vi "niDTS WLAN Rx Test UTIL Static Default Parameters.vi"(10 "Standard":T2 caption="802.11 Standard") -> (2 "Static Default Parameters":T1={"Standard"=enum."802.11 n HT", "DSSS Data Rate (Mbps)"=enum."1", "OFDM Data Rate (Mbps)"=enum."54", "MCS Index"=7, "N Spatial Streams"=1, "Chains"=[TRUE, FALSE, FALSE, FALSE], "Bandwidth (Hz)"=enum."20 MHz", "Channel"=1, "Power (dBm)"=0.0, "Guard Interval"=enum."SHORT", "FEC Coding"=enum."LDPC", "16 symbols"=TRUE, "Payload Length (bytes)"=1500, "Idle Interval (s)"=0.0001, "External Attenuation (dB)"=[0.0, 0.0, 0.0, 0.0], "RX Measurement Parameters"={"Number of Packets"=1000, "MacAddress"="FF:FF:FF:FF:FF:FF"}} {"Idle Interval (s)" format="%_3p"})   [LabVIEW 2015, in "niDTS WLAN.lvlib"]
uses:
  niDTS WLAN.lvlib
  Includes/niDTS WLAN INC Standard.ctl
  Includes/niDTS WLAN Rx Test INC Parameters.ctl
  Includes/niDTS WLAN INC DSSS Data Rate.ctl
  Includes/niDTS WLAN INC OFDM Data Rate.ctl
  Includes/niDTS WLAN INC CH BW.ctl
  Includes/niDTS WLAN INC GI.ctl
  Includes/niDTS WLAN INC FEC Coding.ctl
  Includes/niDTS WLAN INC RX Measurement Parameters.ctl
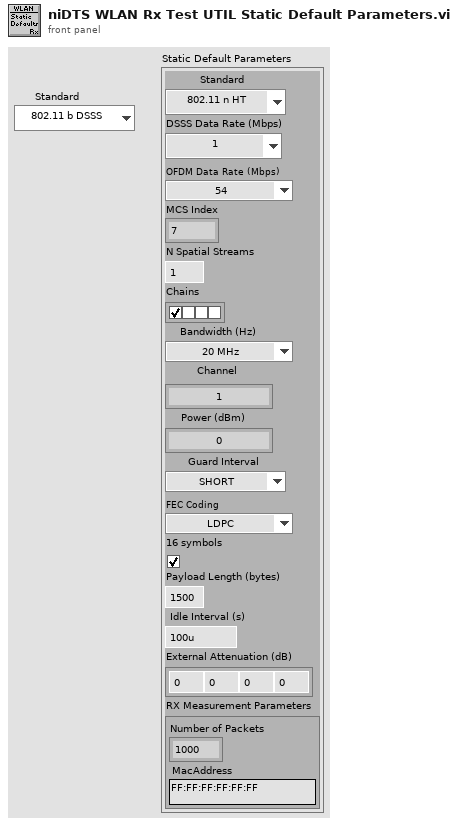
[diagram p1: front panel]
types:
  T1 = typedef "niDTS WLAN.lvlib/niDTS WLAN Rx Test INC Parameters.ctl" = cluster{"Standard":T2, "DSSS Data Rate (Mbps)":T3, "OFDM Data Rate (Mbps)":T4, "MCS Index":i32, "N Spatial Streams":i32, "Chains":bool[], "Bandwidth (Hz)":T5, "Channel":i32, "Power (dBm)":dbl, "Guard Interval":T6, "FEC Coding":T7, "16 symbols":bool, "Payload Length (bytes)":i32, "Idle Interval (s)":dbl, "External Attenuation (dB)":dbl[], "RX Measurement Parameters":T8}
  T2 = typedef "niDTS WLAN.lvlib/niDTS WLAN INC Standard.ctl" = enum16{"802.11 b DSSS", "802.11 a/g OFDM", "802.11 n HT", "802.11 ac VHT"}
  T3 = typedef "niDTS WLAN.lvlib/niDTS WLAN INC DSSS Data Rate.ctl" = enum16{"1", "2", "5.5", "11"}
  T4 = typedef "niDTS WLAN.lvlib/niDTS WLAN INC OFDM Data Rate.ctl" = enum16{"6", "9", "12", "18", "24", "36", "48", "54"}
  T5 = typedef "niDTS WLAN.lvlib/niDTS WLAN INC CH BW.ctl" = enum16{"20 MHz", "40 MHz", "80 MHz", "160 MHz"}
  T6 = typedef "niDTS WLAN.lvlib/niDTS WLAN INC GI.ctl" = enum16{"LONG", "SHORT"}
  T7 = typedef "niDTS WLAN.lvlib/niDTS WLAN INC FEC Coding.ctl" = enum16{"BCC", "LDPC"}
  T8 = typedef "niDTS WLAN.lvlib/niDTS WLAN INC RX Measurement Parameters.ctl" = cluster{"Number of Packets":i32, "MacAddress":string}
  T9 = typedef "niDTS WLAN.lvlib/niDTS WLAN INC Type.ctl" = enum16{"b - 1 Mbps", "b - 2 Mbps", "b - 5.5 Mbps", "b - 11 Mbps", "ag - 6 Mbps", "ag - 9 Mbps", "ag - 12 Mbps", "ag - 18 Mbps", "ag - 24 Mbps", "ag - 36 Mbps", "ag - 48 Mbps", "ag - 54 Mbps", "n - MCS0", "n - MCS1", "n - MCS2", "n - MCS3", "n - MCS4", "n - MCS5", "n - MCS6", "n - MCS7", "n - MCS8", "n - MCS9", "n - MCS10", "n - MCS11", "n - MCS12", "n - MCS13", "n - MCS14", "n - MCS15", "n - MCS16", "n - MCS17", "n - MCS18", "n - MCS19", "n - MCS20", "n - MCS21", "n - MCS22", "n - MCS23", "n - MCS24", "n - MCS25", "n - MCS26", "n - MCS27", "n - MCS28", "n - MCS29", "n - MCS30", "n - MCS31", "ac - MCS0 -1", "ac - MCS1 -1", "ac - MCS2 -1", "ac - MCS3 -1", "ac - MCS4 -1", "ac - MCS5 -1", "ac - MCS6 -1", "ac - MCS7 -1", "ac - MCS8 -1", "ac - MCS9 -1", "ac - MCS0 -2", "ac - MCS1 -2", "ac - MCS2 -2", "ac - MCS3 -2", "ac - MCS4 -2", "ac - MCS5 -2", "ac - MCS6 -2", "ac - MCS7 -2", "ac - MCS8 -2", "ac - MCS9 -2", "ac - MCS0 -3", "ac - MCS1 -3", "ac - MCS2 -3", "ac - MCS3 -3", "ac - MCS4 -3", "ac - MCS5 -3", "ac - MCS6 -3", "ac - MCS7 -3", "ac - MCS8 -3", "ac - MCS9 -3", "ac - MCS0 -4", "ac - MCS1 -4", "ac - MCS2 -4", "ac - MCS3 -4", "ac - MCS4 -4", "ac - MCS5 -4", "ac - MCS6 -4", "ac - MCS7 -4", "ac - MCS8 -4", "ac - MCS9 -4"}
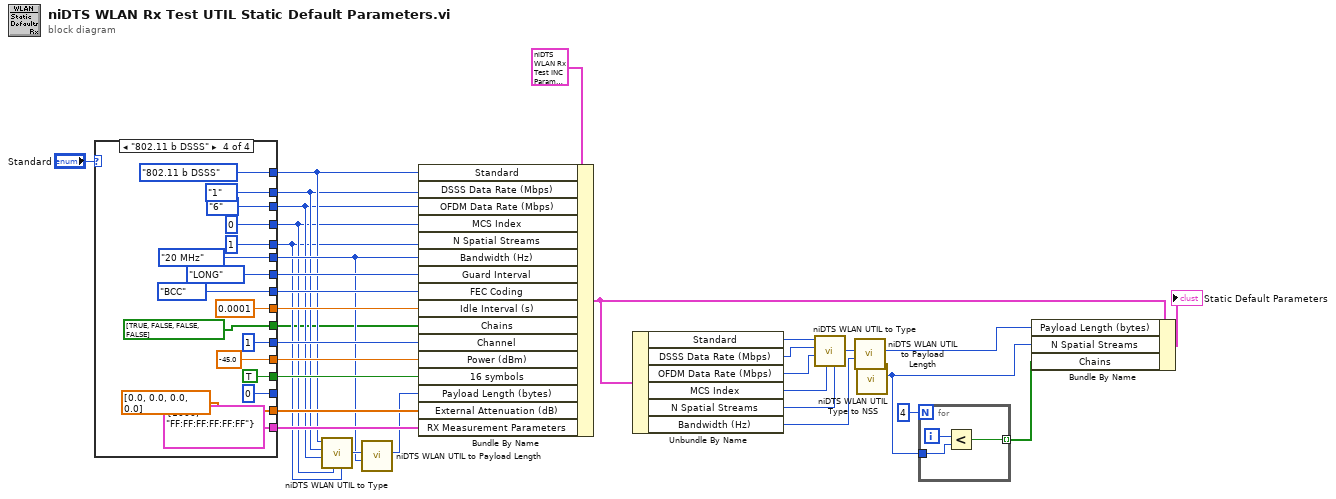
[diagram p0: block diagram]
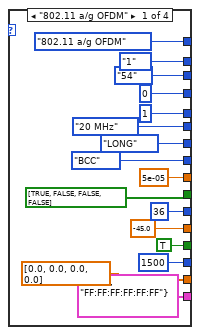
[diagram p2: hidden frame]
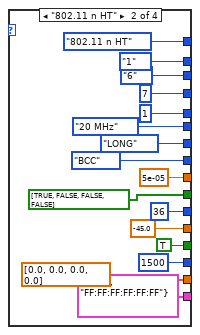
[diagram p3: hidden frame]
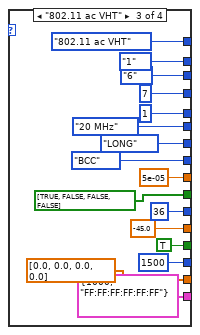
[diagram p4: hidden frame]
diagram:
  n1 = case shown="\"802.11 b DSSS\"" "Standard" {
    tunnel: [niDTS_WLAN_INC_Standard."802.11 a/g OFDM" ("Standard") niDTS_WLAN_INC_Standard."802.11 n HT" ("Standard") niDTS_WLAN_INC_Standard."802.11 ac VHT" ("Standard") niDTS_WLAN_INC_Standard."802.11 b DSSS" ("Standard")] -> w22
    tunnel: [niDTS_WLAN_INC_DSSS_Data_Rate."1" ("DSSS Data Rate (Mbps)") niDTS_WLAN_INC_DSSS_Data_Rate."1" ("DSSS Data Rate (Mbps)") niDTS_WLAN_INC_DSSS_Data_Rate."1" ("DSSS Data Rate (Mbps)") niDTS_WLAN_INC_DSSS_Data_Rate."1" ("DSSS Data Rate (Mbps)")] -> w21
    tunnel: [niDTS_WLAN_INC_OFDM_Data_Rate."54" ("OFDM Data Rate (Mbps)") niDTS_WLAN_INC_OFDM_Data_Rate."6" ("OFDM Data Rate (Mbps)") niDTS_WLAN_INC_OFDM_Data_Rate."6" ("OFDM Data Rate (Mbps)") niDTS_WLAN_INC_OFDM_Data_Rate."6" ("OFDM Data Rate (Mbps)")] -> w20
    tunnel: [0 ("MCS Index") 7 ("MCS Index") 7 ("MCS Index") 0 ("MCS Index")] -> w19
    tunnel: [1 ("N spatial streams") 1 ("N spatial streams") 1 ("N spatial streams") 1 ("N spatial streams")] -> w18
    tunnel: [niDTS_WLAN_INC_CH_BW."20 MHz" ("BandWidth (Hz)") niDTS_WLAN_INC_CH_BW."20 MHz" ("BandWidth (Hz)") niDTS_WLAN_INC_CH_BW."20 MHz" ("BandWidth (Hz)") niDTS_WLAN_INC_CH_BW."20 MHz" ("BandWidth (Hz)")] -> w23
    tunnel: [niDTS_WLAN_INC_GI."LONG" ("Gard Interval") niDTS_WLAN_INC_GI."LONG" ("Gard Interval") niDTS_WLAN_INC_GI."LONG" ("Gard Interval") niDTS_WLAN_INC_GI."LONG" ("Gard Interval")] -> w32
    tunnel: [niDTS_WLAN_INC_FEC_Coding."BCC" ("FEC Coding") niDTS_WLAN_INC_FEC_Coding."BCC" ("FEC Coding") niDTS_WLAN_INC_FEC_Coding."BCC" ("FEC Coding") niDTS_WLAN_INC_FEC_Coding."BCC" ("FEC Coding")] -> w31
    tunnel: [5e-05 ("idle interval") 5e-05 ("idle interval") 5e-05 ("idle interval") 0.0001 ("idle interval")] -> w30
    tunnel: [36 ("Channel") 36 ("Channel") 36 ("Channel") 1 ("Channel")] -> w29
    tunnel: [-45.0 ("Power") -45.0 ("Power") -45.0 ("Power") -45.0 ("Power")] -> w28
    tunnel: [TRUE ("16 symbols") TRUE ("16 symbols") TRUE ("16 symbols") TRUE ("16 symbols")] -> w27
    tunnel: [1500 ("payload length bytes") 1500 ("payload length bytes") 1500 ("payload length bytes") 0 ("payload length bytes")] -> _
    tunnel: [dbl[] [0.0, 0.0, 0.0, 0.0] dbl[] [0.0, 0.0, 0.0, 0.0] dbl[] [0.0, 0.0, 0.0, 0.0] dbl[] [0.0, 0.0, 0.0, 0.0]] -> w26
    tunnel: [T8 {"Number of Packets"=1000, "MacAddress"="FF:FF:FF:FF:FF:FF"} ("RX Measurement Parameters") T8 {"Number of Packets"=1000, "MacAddress"="FF:FF:FF:FF:FF:FF"} ("RX Measurement Parameters") T8 {"Number of Packets"=1000, "MacAddress"="FF:FF:FF:FF:FF:FF"} ("RX Measurement Parameters") T8 {"Number of Packets"=1000, "MacAddress"="FF:FF:FF:FF:FF:FF"} ("RX Measurement Parameters")] -> w25
    tunnel: [bool[] [TRUE, FALSE, FALSE, FALSE] ("Chains") bool[] [TRUE, FALSE, FALSE, FALSE] ("Chains") bool[] [TRUE, FALSE, FALSE, FALSE] ("Chains") bool[] [TRUE, FALSE, FALSE, FALSE] ("Chains")] -> w5
    frame "802.11 a/g OFDM" {
    }
    frame "802.11 n HT" {
    }
    frame "802.11 ac VHT" {
    }
    frame "802.11 b DSSS" {
    }
  }
  n2 = call "niDTS WLAN UTIL to Type.vi"("N_SS"=w18, "MCS"=w19, "OFDM Data Rate (Mbps)"=w20, "DSSS Data Rate (Mbps)"=w21, "Standard"=w22) -> ("WLAN Type"=w24:T9)  [unwired: 6 in]
  n3 = call "niDTS WLAN UTIL to Payload Length.vi"("CH BW"=w23, "WLAN Type"=w24) -> ("Payload Length"=w17:i32)  [unwired: 9 in]
  n4 = Bundle By Name(cluster=T1 {"Standard"=enum."802.11 b DSSS", "DSSS Data Rate (Mbps)"=enum."1", "OFDM Data Rate (Mbps)"=enum."6", "MCS Index"=0, "N Spatial Streams"=0, "Chains"=[TRUE, FALSE, FALSE, FALSE], "Bandwidth (Hz)"=enum."20 MHz", "Channel"=0, "Power (dBm)"=0.0, "Guard Interval"=enum."LONG", "FEC Coding"=enum."BCC", "16 symbols"=FALSE, "Payload Length (bytes)"=0, "Idle Interval (s)"=0.0, "External Attenuation (dB)"=[0.0, 0.0, 0.0, 0.0], "RX Measurement Parameters"={"Number of Packets"=0, "MacAddress"="FF:FF:FF:FF:FF:FF"}} ("Parameters"), "Standard"=w22, "DSSS Data Rate (Mbps)"=w21, "OFDM Data Rate (Mbps)"=w20, "MCS Index"=w19, "N Spatial Streams"=w18, "Bandwidth (Hz)"=w23, "Guard Interval"=w32, "FEC Coding"=w31, "Idle Interval (s)"=w30, "Chains"=w5, "Channel"=w29, "Power (dBm)"=w28, "16 symbols"=w27, "Payload Length (bytes)"=w17, "External Attenuation (dB)"=w26, "RX Measurement Parameters"=w25) -> (w7:T1)
  n5 = Unbundle By Name(w7) -> ("Standard"=w8:T2, "DSSS Data Rate (Mbps)"=w10:T3, "OFDM Data Rate (Mbps)"=w11:T4, "MCS Index"=w12:i32, "N Spatial Streams"=w13:i32, "Bandwidth (Hz)"=w14:T5)
  n6 = call "niDTS WLAN UTIL to Type.vi"("N_SS"=w13, "MCS"=w12, "OFDM Data Rate (Mbps)"=w11, "DSSS Data Rate (Mbps)"=w10, "Standard"=w8) -> ("WLAN Type"=w4:T9)  [unwired: 6 in]
  n7 = call "niDTS WLAN UTIL to Payload Length.vi"("CH BW"=w14, "WLAN Type"=w4) -> ("Payload Length"=w9:i32)  [unwired: 9 in]
  n8 = call "niDTS WLAN UTIL Type to NSS.vi"("WLAN Type"=w4) -> ("NSS"=w2:i32)  [unwired: 10 in]
  n9 = for {
    N: 4 -> [_]
    tunnel: w2 -> [w98]
    tunnel: [w97] -> w1 mode=indexing
    i -> [w99]
    n10 = Less?(x=w99, y=w98) -> (x < y?=w97:bool)
  }
  n11 = Bundle By Name(cluster=w7, "Payload Length (bytes)"=w9, "N Spatial Streams"=w2, "Chains"=w1) -> (→"Static Default Parameters":T1)
